vi "可见度.vi"(1 "输入数组":dbl[][](array[numeric])) -> (0 "可见度":dbl)   [LabVIEW 2018]
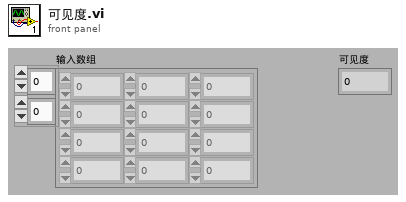
[diagram p1: front panel]
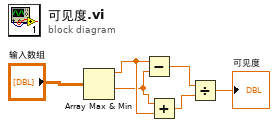
[diagram p0: block diagram]
diagram:
  n1 = Array Max & Min(array="输入数组") -> (max value=w5:dbl, min value=w4:dbl)  [unwired: 2 out]
  n2 = Subtract(x=w5, y=w4) -> (x-y=w2:dbl)
  n3 = Add(x=w4, y=w5) -> (x+y=w3:dbl)
  n4 = Divide(x=w2, y=w3) -> (x/y=→"可见度":dbl)
